vi "target distance.vi"(11 "Blobs":T1) -> (3 "Blobs + distance":T1)   [LabVIEW 2014]
uses:
  target type.ctl
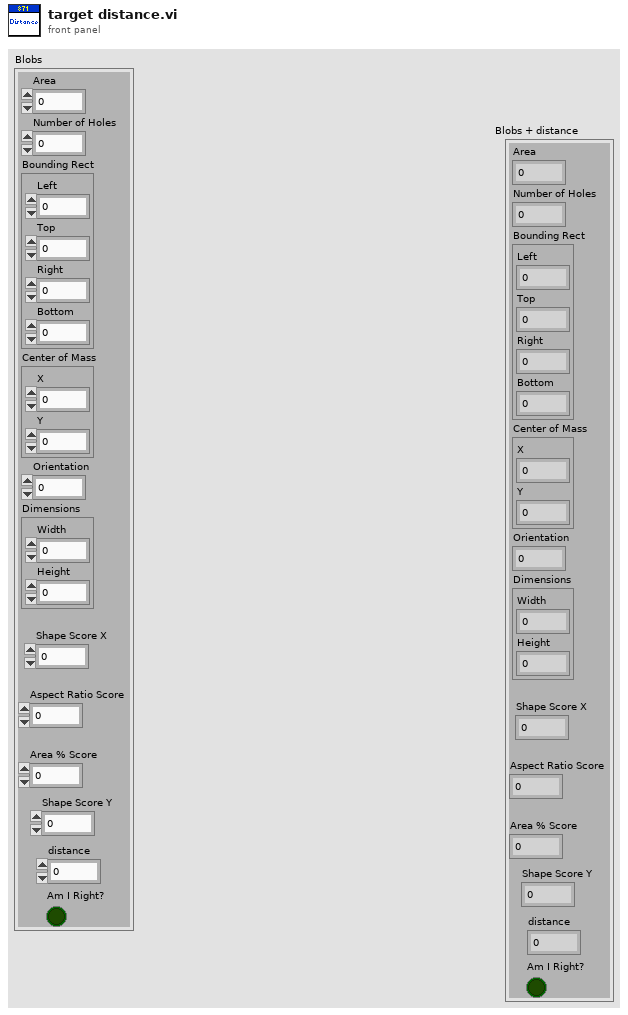
[diagram p1: front panel]
types:
  T1 = typedef "target type.ctl" = cluster{"Area":dbl, "Number of Holes":dbl, "Bounding Rect":cluster{"Left":dbl, "Top":dbl, "Right":dbl, "Bottom":dbl}, "Center of Mass":cluster{"X":dbl, "Y":dbl}, "Orientation":dbl, "Dimensions":cluster{"Width":dbl, "Height":dbl}, "Shape Score X":dbl, "Aspect Ratio Score":dbl, "Area % Score":dbl, "Shape Score Y":dbl, "Am I Right?":bool, "distance":dbl}
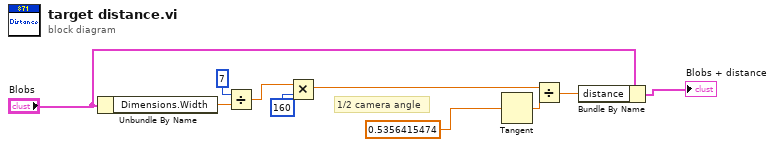
[diagram p0: block diagram]
diagram:
  # "1/2 camera angle"
  n1 = Unbundle By Name("Blobs") -> ("Dimensions.Width"=w10:dbl)
  n2 = Divide(x=7, y=w10) -> (x/y=w7:dbl)
  n3 = Multiply(x=w7, y=160) -> (x*y=w5:dbl)
  n4 = Tangent(1:0.5356415474) -> (0:w6:dbl)
  n5 = Divide(x=w5, y=w6) -> (x/y=w4:dbl)
  n6 = Bundle By Name(cluster="Blobs", "distance"=w4) -> (→"Blobs + distance":T1)
